vi "daylight savings time adj.vi"(2 "Apply daylight savings time":bool, 7 "Date Time (IN)":T1) -> (8 "Date Time (out)":T1)   [LabVIEW 2011]
doc: "This VI only adjusts for daylight savings time for 2011. It needs modified or adapted for any other year"
uses:
  <vilib>/Utility/miscctls.llb/LVDateTimeRec.ctl
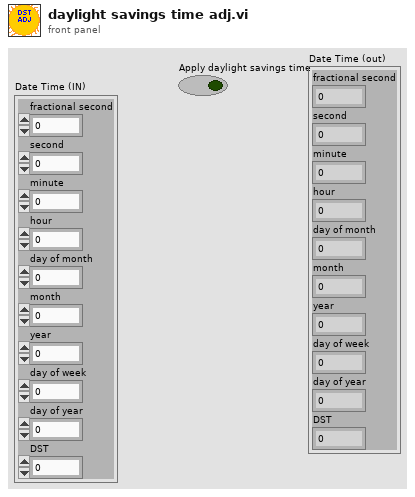
[diagram p1: front panel]
types:
  T1 = typedef "LVDateTimeRec.ctl" = cluster{"fractional second":dbl, "second":i32, "minute":i32, "hour":i32, "day of month":i32, "month":i32, "year":i32, "day of week":i32, "day of year":i32, "DST":i32}
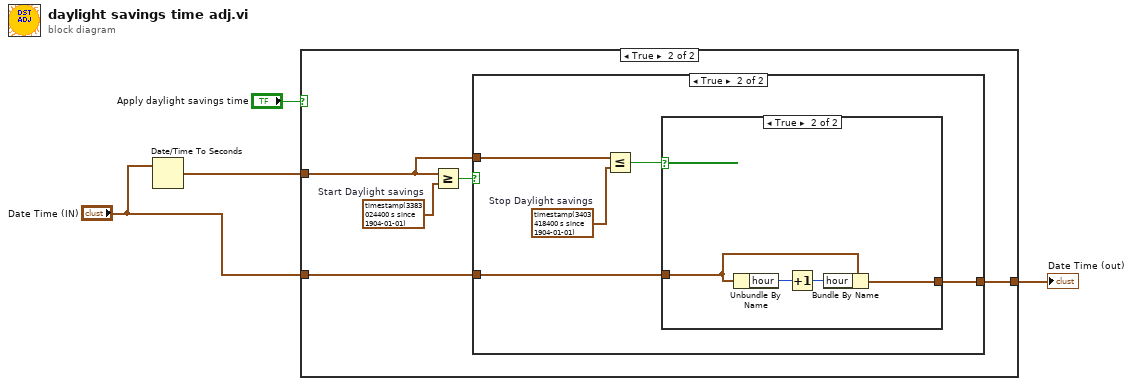
[diagram p0: block diagram]
diagram:
  n1 = Date/Time To Seconds(2:"Date Time (IN)") -> (0:w1:timestamp)  [unwired: 1 in]
  n2 = case shown="True" "Apply daylight savings time" {
    tunnel: w1 -> [_ w8]
    tunnel: [w5 w7] -> w3
    tunnel: "Date Time (IN)" -> [w5 w6]
    frame False {
    }
    frame True {
      w9 = timestamp(3383024400 s since 1904-01-01)  # Start Daylight savings
      n3 = Greater Or Equal?(x=w8, y=w9) -> (x >= y?=w10:bool)
      n4 = case shown="True" w10 {
        tunnel: w8 -> [_ w15]
        tunnel: w6 -> [w11 w13]
        tunnel: [w11 w12] -> w7
        frame False {
        }
        frame True {
          w14 = timestamp(3403418400 s since 1904-01-01)  # Stop Daylight savings
          n5 = Less Or Equal?(x=w15, y=w14) -> (x <= y?=w16:bool)
          n6 = case shown="True" w16 {
            tunnel: w13 -> [w17 w18]
            tunnel: [w17 w19] -> w12
            frame False {
            }
            frame True {
              n7 = Unbundle By Name(w18) -> ("hour"=w21:i32)
              n8 = Increment(x=w21) -> (x+1=w20:i32)
              n9 = Bundle By Name(cluster=w18, "hour"=w20) -> (w19:T1)
            }
          }
        }
      }
    }
  }
  "Date Time (out)" <- w3
